vi "Escalar_x_vector.vi"(10 "Numeric":ext, 11 "Array in":ext[](array[numeric])) -> (3 "Array out":ext[](array[numeric]))   [LabVIEW 2011]
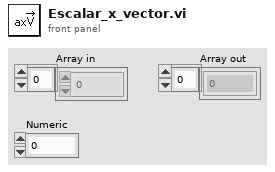
[diagram p1: front panel]
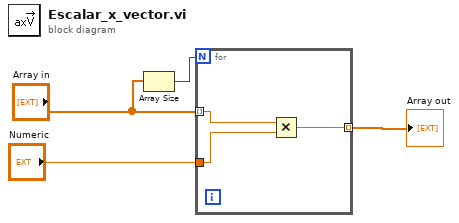
[diagram p0: block diagram]
diagram:
  n1 = Array Size(array="Array in") -> (size(s)=w1:i32)
  n2 = for {
    N: w1 -> [_]
    tunnel: [w7] -> w4 mode=indexing
    tunnel: "Array in" -> [w6] mode=indexing
    tunnel: "Numeric" -> [w5]
    n3 = Multiply(x=w6, y=w5) -> (x*y=w7:ext)
  }
  "Array out" <- w4
